vi "TryLoadGainCorrectionImages.vi"(10 "Pixel Calibration Offset Image":path, 11 "Pixel Calibration Gain Image":path) -> (0 "-Offset flat":sgl[](array[numeric]), 1 "1/Gain flat":sgl[](array[numeric]), 2 "-Offset":sgl[][](array[numeric]), 3 "Normalized 1/Gain":sgl[][](array[numeric]))   [LabVIEW 2011]
panel:
  in  "Negate offset":bool=TRUE
  in  "Invert gain?":bool=TRUE
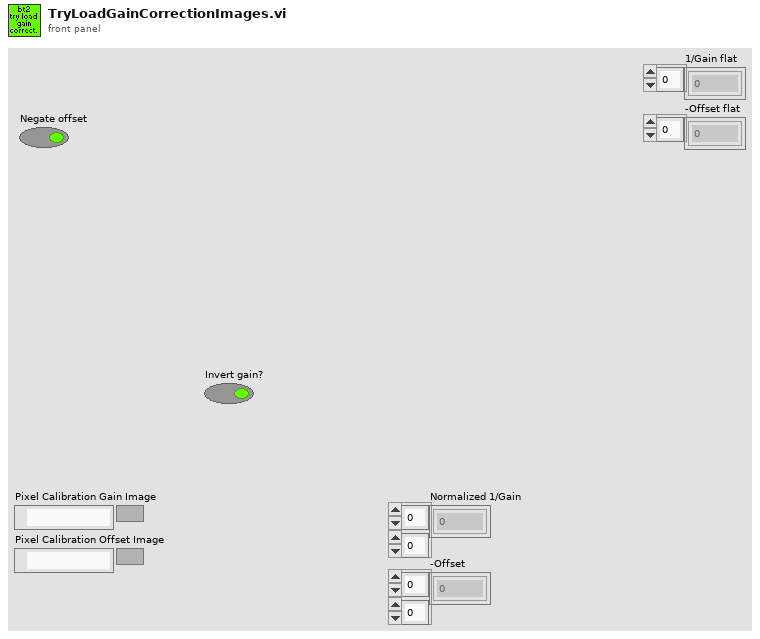
[diagram p1: front panel]
types:
  T1 = enum16{"big-endian, network order", "native, host order", "little-endian"}
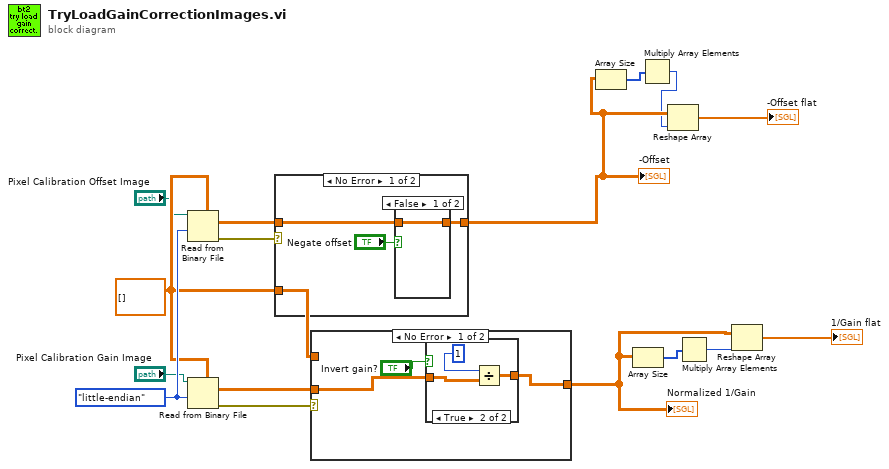
[diagram p0: block diagram]
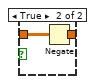
[diagram p2: hidden frame]
diagram:
  w16 = T1."little-endian" ("byte order (0:big-endian, network order)")
  w11 = sgl[][] []
  n1 = Read from Binary File(5:w11, 9:w16, 11:"Pixel Calibration Offset Image") -> (0:w14:errorcluster, 2:w12:sgl[][])  [unwired: 3 in, 2 out]
  n2 = Read from Binary File(5:w11, 9:w16, 11:"Pixel Calibration Gain Image") -> (0:w15:errorcluster, 2:w13:sgl[][])  [unwired: 3 in, 2 out]
  n3 = case shown="No Error" w14 {
    tunnel: [w18 w23] -> w8
    tunnel: w12 -> [w19 _]
    tunnel: w11 -> [_ w23]
    frame No Error {
      n4 = case shown="False" "Negate offset" {
        tunnel: w19 -> [w20 w22]
        tunnel: [w20 w21] -> w18
        frame False {
        }
        frame True {
          n5 = Negate(x=w22) -> (-x=w21:sgl[][])
        }
      }
    }
    frame Error {
    }
  }
  "-Offset" <- w8
  n6 = case shown="No Error" w15 {
    tunnel: w13 -> [w26 _]
    tunnel: [w25 w31] -> w3
    tunnel: w11 -> [_ w31]
    frame No Error {
      n7 = case shown="True" "Invert gain?" {
        tunnel: w26 -> [w27 w30]
        tunnel: [w27 w29] -> w25
        frame False {
        }
        frame True {
          n8 = Divide(x=1, y=w30) -> (x/y=w29:sgl[][])
        }
      }
    }
    frame Error {
    }
  }
  "Normalized 1/Gain" <- w3
  n9 = Array Size(array=w8) -> (size(s)=w7:i32[])
  n10 = Array Size(array=w3) -> (size(s)=w5:i32[])
  n11 = Multiply Array Elements(1:w7) -> (0:w6:i32)
  n12 = Reshape Array(w8, w6) -> (→"-Offset flat":sgl[])
  n13 = Multiply Array Elements(1:w5) -> (0:w4:i32)
  n14 = Reshape Array(w3, w4) -> (→"1/Gain flat":sgl[])
